vi "超标留样启动流程.vi"   [LabVIEW 2016, in "德润DR803F超标留样.lvlib"]
types:
  T1 = cluster{"工作状态":u16, "工作进程":u16, "仪器时间":timestamp, "采样模式":u16, "当前瓶号":dbl, "采样瓶数":dbl, "每瓶采样次数":dbl, "当前瓶已采次数":dbl, "当前瓶采样量":dbl, "采样量定量":dbl, "采样量比例":dbl, "瞬时流量":dbl, "累积流量":dbl, "外置泵状态":dbl, "采样泵状态":dbl, "采样泵方向":dbl, "采样阀":dbl, "采样瓶转盘":dbl, "排水阀":dbl, "清洗泵":dbl, "清洗管工作":dbl, "清洗管电源":dbl, "清洗管运行方向":dbl, "门状态":u16, "采水管有水检测":dbl}
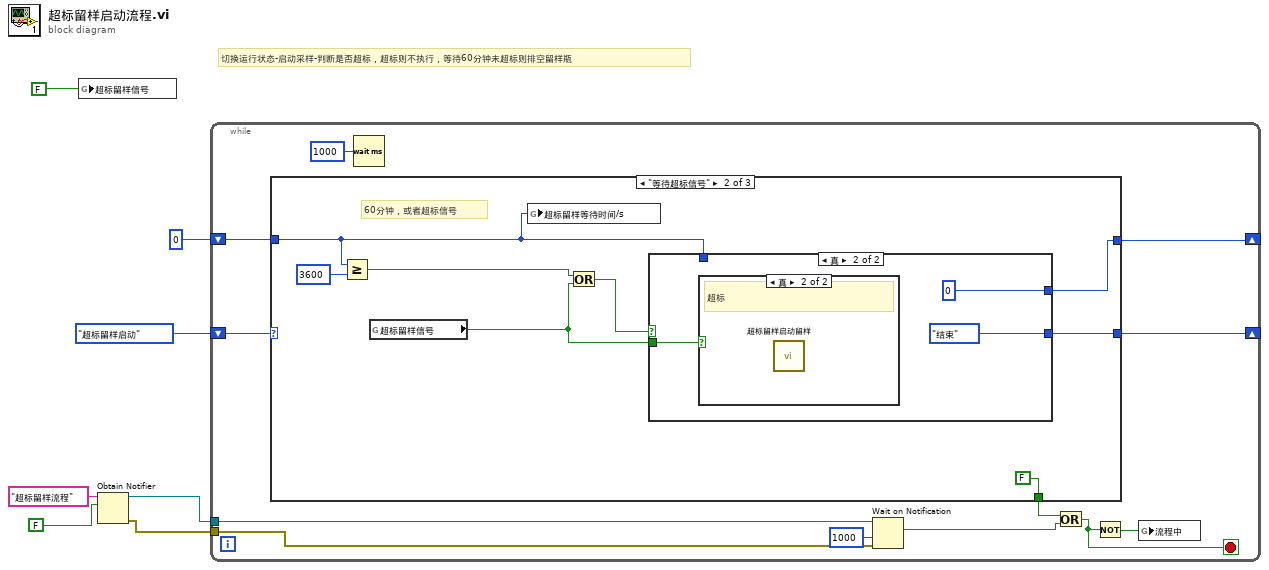
[diagram p0: block diagram]
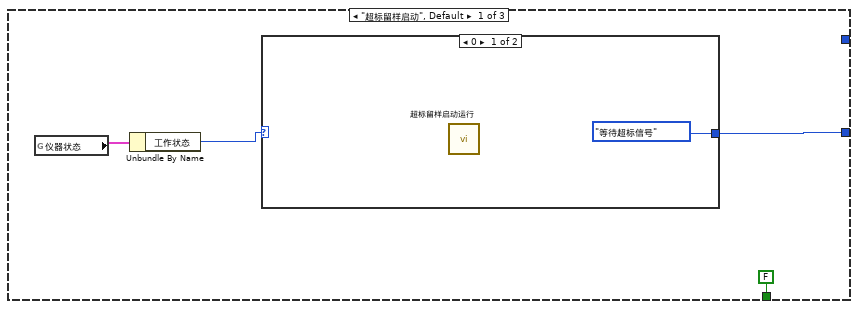
[diagram p2: hidden frame]
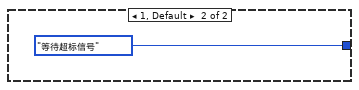
[diagram p3: hidden frame]
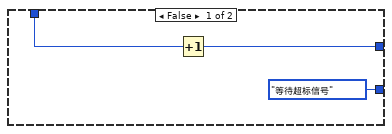
[diagram p4: hidden frame]
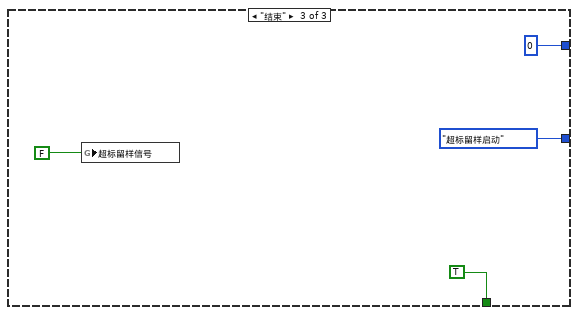
[diagram p6: hidden frame]
diagram:
  # "切换运行状态-启动采样-判断是否超标，超标则不执行，等待60分钟未超标则排空留样瓶"
  n1 = global write "超标留样全局.vi" "超标留样信号"(FALSE ("采样完成")) -> ()
  n2 = Obtain Notifier(name (unnamed)="超标留样流程" ("名称（未命名）"), notification data type=FALSE ("采样完成")) -> (notifier out=w3:refnum<notifier>, error out=w2:errorcluster)  [unwired: 2 in, 1 out]
  n3 = while {
    shift-right: [w9] -> _
    shift-left: enum16{"超标留样启动", "等待超标信号", "结束"}."超标留样启动" -> [w19]
    shift-right: [w16] -> _
    shift-left: 0 -> [w17]
    tunnel: w3 -> [w15]
    tunnel: w2 -> [w14]
    stop <- w12 stop-if-true
    n4 = case shown="\"等待超标信号\"" w19 {
      tunnel: w17 -> [_ w26 _]
      tunnel: [_ w31 0] -> w16
      tunnel: [w20 w29 enum16{"超标留样启动", "等待超标信号", "结束"}."超标留样启动"] -> w9
      tunnel: [FALSE FALSE TRUE] -> w8
      frame "超标留样启动", Default {
        n5 = global read "超标留样全局.vi" "仪器状态"() -> (w23:T1)
        n6 = Unbundle By Name(w23) -> ("工作状态"=w21:u16)
        n7 = case shown="0" w21 {
          tunnel: [enum16{"超标留样启动", "等待超标信号", "结束"}."等待超标信号" enum16{"超标留样启动", "等待超标信号", "结束"}."等待超标信号"] -> w20
          frame 0 {
            n8 = call "超标留样启动运行.vi"() -> ()  [unwired: 11 in, 1 out]
          }
          frame 1, Default {
          }
        }
      }
      frame "等待超标信号" {
        # "60分钟，或者超标信号"
        n9 = Greater Or Equal?(x=w26, y=3600) -> (x >= y?=w32:bool)
        n10 = global read "超标留样全局.vi" "超标留样信号"() -> (w28:bool)
        n11 = global write "超标留样全局.vi" "超标留样等待时间/s"(w26) -> ()
        n12 = Or(x=w32, y=w28) -> (x .or. y?=w30:bool)
        n13 = case shown="真" w30 {
          tunnel: [enum16{"超标留样启动", "等待超标信号", "结束"}."等待超标信号" enum16{"超标留样启动", "等待超标信号", "结束"}."结束"] -> w29
          tunnel: w26 -> [w36 _]
          tunnel: [w35 0] -> w31
          tunnel: w28 -> [_ w37]
          frame False {
            n14 = Increment(x=w36) -> (x+1=w35:i32)
          }
          frame True {
            n15 = case shown="真" w37 {
              frame False {
                # "超时但不超标"
              }
              frame True {
                # "超标"
                n16 = call "超标留样启动留样.vi"() -> ()  [unwired: 11 in, 1 out]
              }
            }
          }
        }
      }
      frame "结束" {
        n17 = global write "超标留样全局.vi" "超标留样信号"(FALSE ("采样完成")) -> ()
      }
    }
    n18 = Wait (ms)(milliseconds to wait=u32 1000 ("等待时间（毫秒）")) -> ()  [unwired: 1 out]
    n19 = Wait on Notification(notifier=w15, timeout in ms (-1)=1000 ("超时毫秒(-1)"), error in (no error)=w14) -> (notification=w11:bool)  [unwired: 1 in, 3 out]
    n20 = Or(x=w8, y=w11) -> (x .or. y?=w12:bool)
    n21 = Not(x=w12) -> (.not. x?=w10:bool)
    n22 = global write "超标留样全局.vi" "流程中"(w10) -> ()
  }
